vi "Status.vi"(8 "error in (no error)":errorcluster, 9 "totalscans":u32 caption="Total Scans", 10 "scan#":u32 caption="Scan Number", 11 "Scanner.lvclass in":refnum<class "Scanner.lvclass">) -> (0 "error out":errorcluster, 2 "scanprogress":string caption="Scan Progress", 3 "Scanner.lvclass out":refnum<class "Scanner.lvclass">)   [LabVIEW 2009, in "Scanner.lvclass"]
doc: "(Dynamic) Return a text status message reflecting the current state of this Scanner."
uses:
  Scanner.lvclass
  Scanner.lvclass/Scanner.ctl
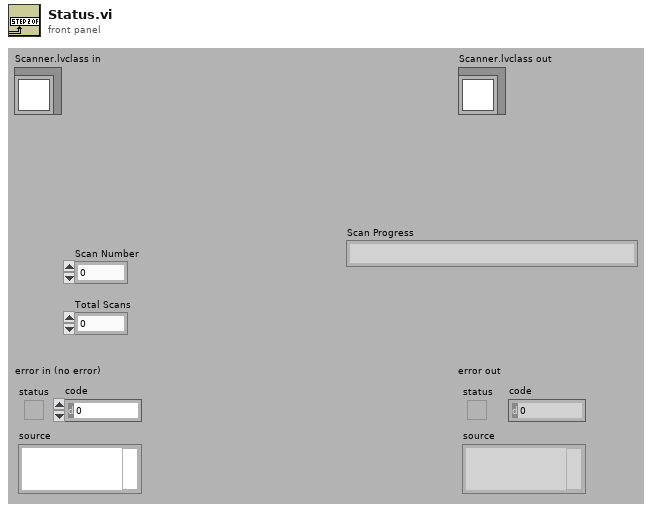
[diagram p1: front panel]
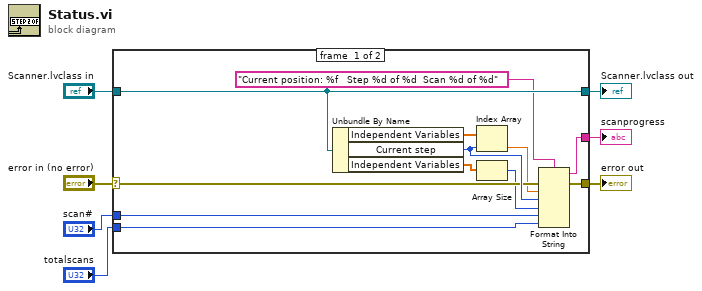
[diagram p0: block diagram]
diagram:
  n1 = case shown="No Error" "error in (no error)" {
    selector: "error in (no error)" -> [w14 w20]
    tunnel: [w13 w20] -> w6
    tunnel: [w19 w21] -> w4
    tunnel: "Scanner.lvclass in" -> [w19 w21]
    tunnel: [w11 _] -> w3
    tunnel: "totalscans" -> [w10 _]
    tunnel: "scan#" -> [w9 _]
    frame #0 {
      n2 = Unbundle By Name(w19) -> ("Independent Variables"=w18:dbl[], "Current step"=w16:u32, "Independent Variables"=w15:dbl[])
      n3 = Index Array(array=w18, index=w16) -> (element=w12:dbl)
      n4 = Array Size(array=w15) -> (size(s)=w8:i32)
      n5 = Format Into String(format string="Current position: %f   Step %d of %d  Scan %d of %d", error in=w14, w12, w16, w8, w9, w10) -> (resulting string=w11:string, error out=w13:errorcluster)  [unwired: 1 in]
    }
    frame #1 {
    }
  }
  "error out" <- w6
  "Scanner.lvclass out" <- w4
  "scanprogress" <- w3
